vi "create.vi"(10 "Workspace":T1) -> (2 "Workspace":refnum<class "workspace.lvclass">)   [LabVIEW 2020, in "nominal types.lvlib" / "workspace.lvclass"]
uses:
  workspace.lvclass
  workspace.lvclass/workspace.ctl
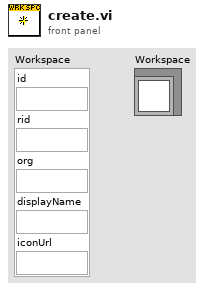
[diagram p1: front panel]
types:
  T1 = cluster{"id":string, "rid":string, "org":string, "displayName":string, "iconUrl":string}
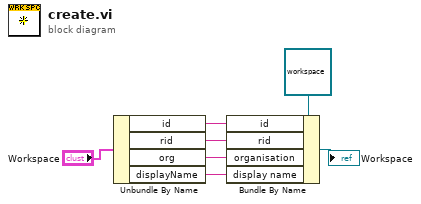
[diagram p0: block diagram]
diagram:
  n1 = Unbundle By Name("Workspace") -> ("id"=w5:string, "rid"=w4:string, "org"=w3:string, "displayName"=w2:string)
  n2 = Bundle By Name(cluster=refnum<class "workspace.lvclass"> refnum ("nominal types.lvlib:workspace.lvclass"), "id"=w5, "rid"=w4, "organisation"=w3, "display name"=w2) -> (→"Workspace":refnum<class "workspace.lvclass">)
